vi "ASI_Move.vi"(8 "error in (no error)":errorcluster, 9 "Position [mm]":dbl, 10 "Axis":string(combo), 11 "VISA resource name":refnum<visa-resource-name>) -> (0 "error out":errorcluster, 3 "VISA resource name out":refnum<visa-resource-name>)   [LabVIEW 2011]
panel:
  out "read buffer":string
  out "write buffer":string="M X=1234.5 Y=1234.5"
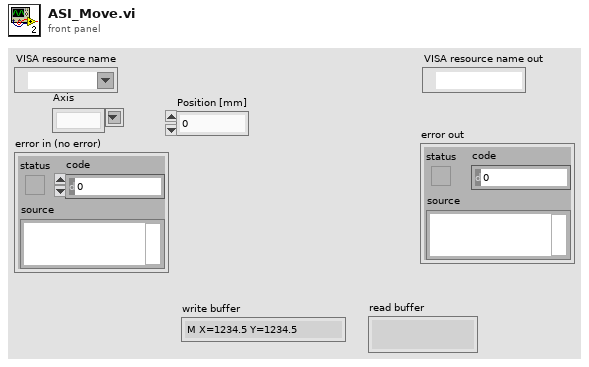
[diagram p1: front panel]
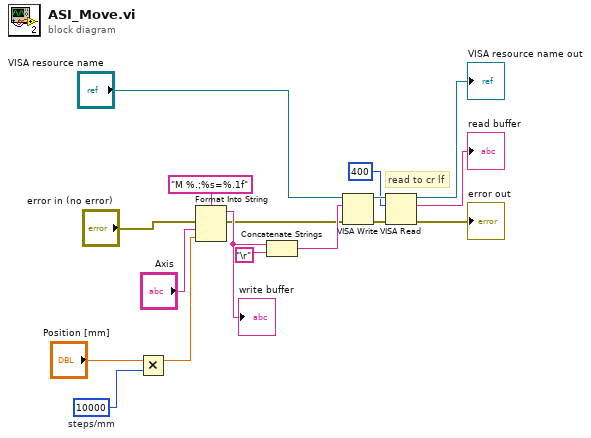
[diagram p0: block diagram]
diagram:
  w1 = 10000  # steps/mm
  # "read to cr lf"
  n1 = Multiply(x="Position [mm]", y=w1) -> (x*y=w2:dbl)
  n2 = Format Into String(format string="M %.;%s=%.1f", error in="error in (no error)", "Axis", w2) -> (resulting string=w7:string, error out=w4:errorcluster)  [unwired: 1 in]
  "write buffer" <- w7
  n3 = Concatenate Strings(w7, "\r") -> (w17:string)
  n4 = VISA Write(VISA resource name="VISA resource name", write buffer=w17, error in (no error)=w4) -> (VISA resource name out=w15:refnum<visa-resource-name>, error out=w12:errorcluster)  [unwired: 1 out]
  n5 = VISA Read(VISA resource name=w15, byte count=u32 400, error in (no error)=w12) -> (VISA resource name out=→"VISA resource name out":refnum<visa-resource-name>, read buffer=→"read buffer":string, error out=→"error out":errorcluster)  [unwired: 1 out]
